vi "Get Callback User Events.vi"(11 "SourceGrid in":refnum<class "SourceGrid.lvclass">) -> (2 "Callback User Events":cluster{"onGridClick":refnum<user-event>}, 3 "SourceGrid out":refnum<class "SourceGrid.lvclass">)   [LabVIEW 2024, in "SourceGrid.lvlib" / "SourceGrid.lvclass"]
uses:
  SourceGrid.lvclass
  MouseEventArgs/MouseEventArgs.lvclass
  SourceGrid.lvclass/SourceGrid.ctl
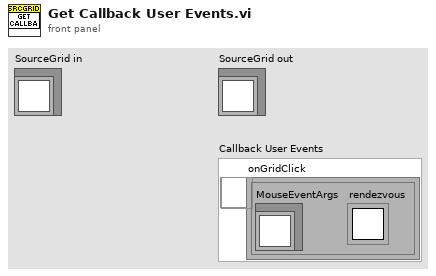
[diagram p1: front panel]
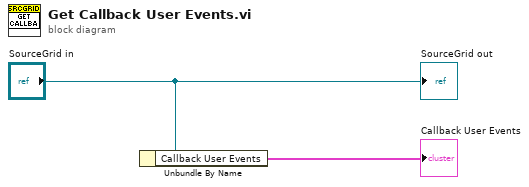
[diagram p0: block diagram]
diagram:
  n1 = Unbundle By Name("SourceGrid in") -> ("Callback User Events"=→"Callback User Events":cluster{"onGridClick":refnum<user-event>})
  "SourceGrid out" <- "SourceGrid in"
